vi "MultiThreadExample.vi"() -> ()   [LabVIEW 2021]
panel:
  out "element":i32
  out "# elements in queue":i32
  in  "Queue Status":bool
  in  "Stop":bool
  out "Numeric":i32
  in  "Enqeue":bool
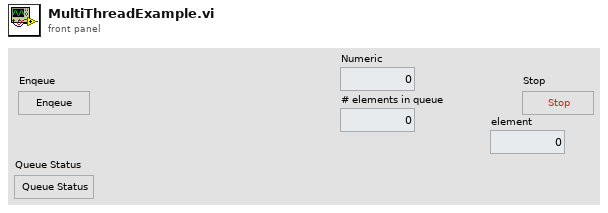
[diagram p1: front panel]
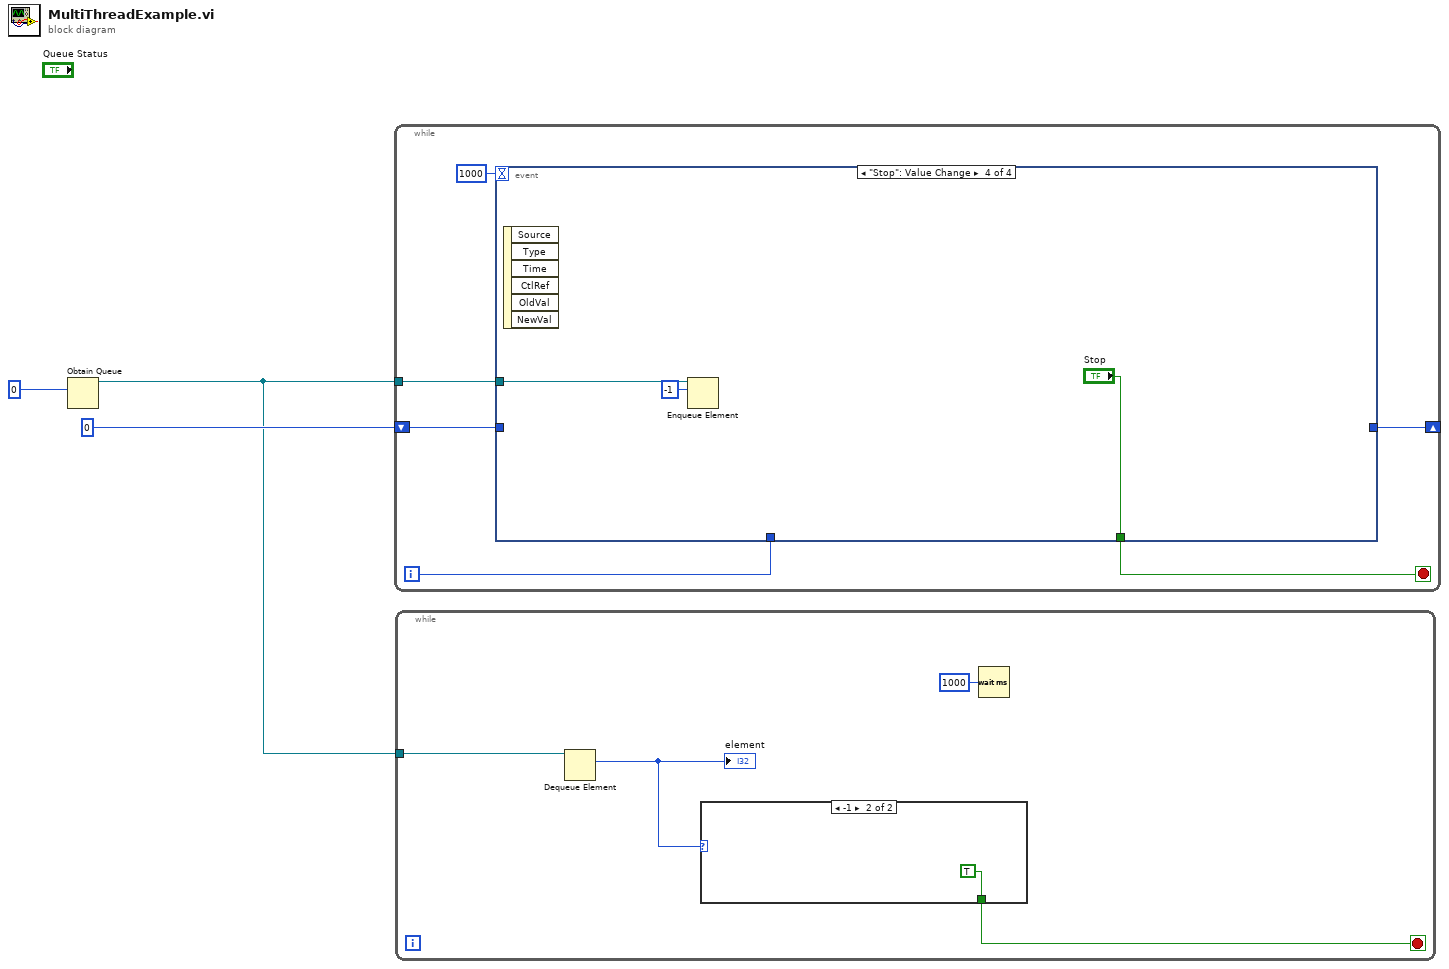
[diagram p0: block diagram]
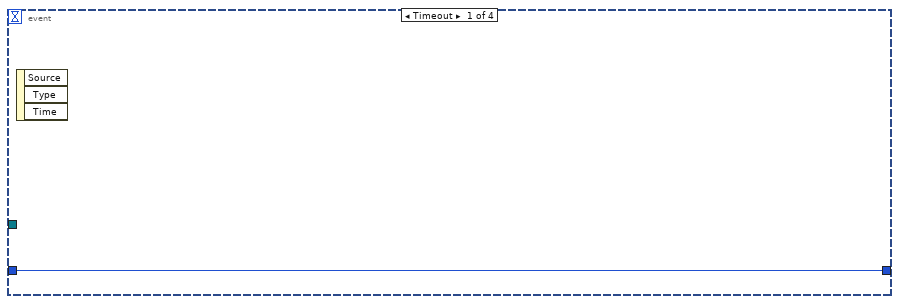
[diagram p3: hidden frame]
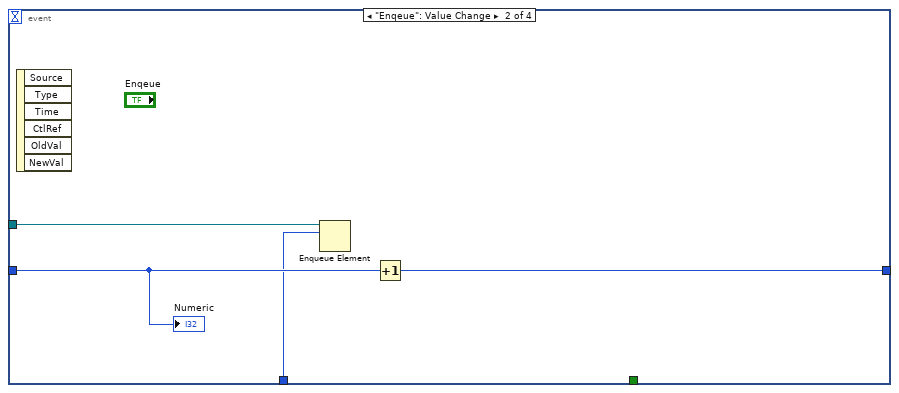
[diagram p4: hidden frame]
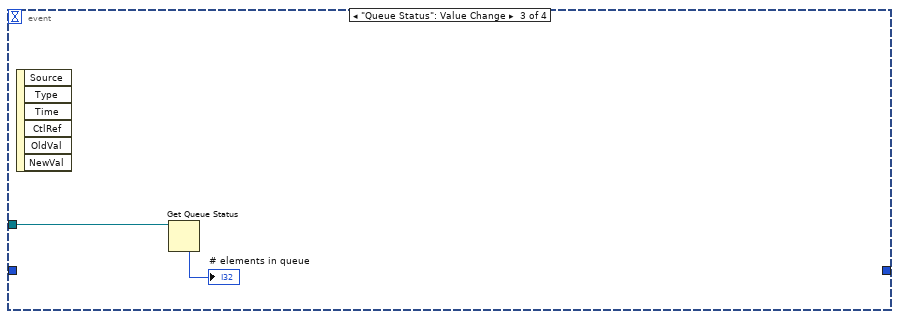
[diagram p5: hidden frame]
diagram:
  n1 = Obtain Queue(element data type=0) -> (queue out=w1:refnum<queue>)  [unwired: 4 in, 2 out]
  n2 = while {
    tunnel: w1 -> [w9]
    shift-right: [w7] -> _
    shift-left: 0 -> [w8]
    i -> [w5]
    stop <- w6 stop-if-true
    n3 = event shown="[3] \"Stop\": Value Change" {
      selector: _ -> [_ _ _ _]
      dyn-events: _ -> [_ _ _ _]
      timeout: 1000 -> [_ _ _ _]
      tunnel: w9 -> [_ w12 w16 w18]
      tunnel: w8 -> [w10 w14 _ _]
      tunnel: [w10 w13 _ _] -> w7
      tunnel: [_ _ _ "Stop"] -> w6
      tunnel: w5 -> [_ w11 _ _]
      event Timeout {
        n4 = event-data() -> ()  [unwired: 1 in, 3 out]
      }
      event "Enqeue": Value Change {
        n5 = event-data() -> ()  [unwired: 1 in, 6 out]
        n6 = Enqueue Element(queue=w12, element=w11) -> ()  [unwired: 2 in, 3 out]
        n7 = Increment(x=w14) -> (x+1=w13:i32)
        "Numeric" <- w14
      }
      event "Queue Status": Value Change {
        n8 = event-data() -> ()  [unwired: 1 in, 6 out]
        n9 = Get Queue Status(queue=w16) -> (# elements in queue=→"# elements in queue":i32)  [unwired: 2 in, 7 out]
      }
      event "Stop": Value Change {
        n10 = event-data() -> ()  [unwired: 1 in, 6 out]
        n11 = Enqueue Element(queue=w18, element=-1) -> ()  [unwired: 2 in, 3 out]
      }
    }
  }
  n12 = while {
    tunnel: w1 -> [w23]
    stop <- w21 stop-if-true
    n13 = Dequeue Element(queue=w23) -> (element=w22:i32)  [unwired: 2 in, 3 out]
    "element" <- w22
    n14 = case shown="-1" w22 {
      tunnel: [_ TRUE] -> w21
      frame Default {
      }
      frame -1 {
      }
    }
    n15 = Wait (ms)(milliseconds to wait=u32 1000) -> ()  [unwired: 1 out]
  }
